vi "11_jednoduchy_trigger.vi"() -> ()   [LabVIEW 2019]
panel:
  in  "Reset Trigger":bool
  out "Hold Trigger":bool
  out "Once Trigger":bool
  out "Waveform Chart":T1(graph)
  in  "stop":bool
  in  "Aktualni hodnota (V)":dbl
  in  "Trigger hodnota (V)":dbl
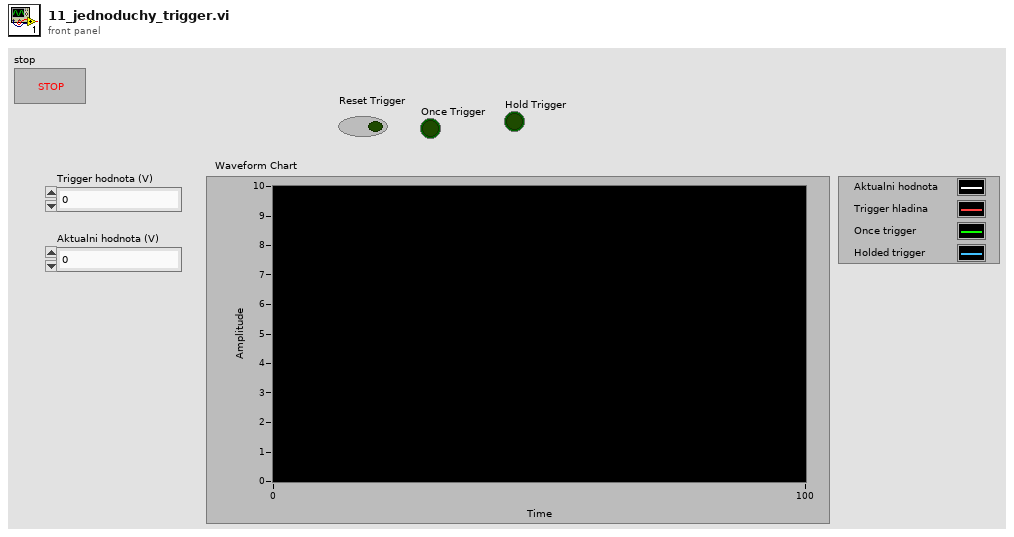
[diagram p1: front panel]
types:
  T1 = cluster{"Aktualni hodnota (V)":dbl, "Trigger hodnota (V)":dbl, i16, i16}
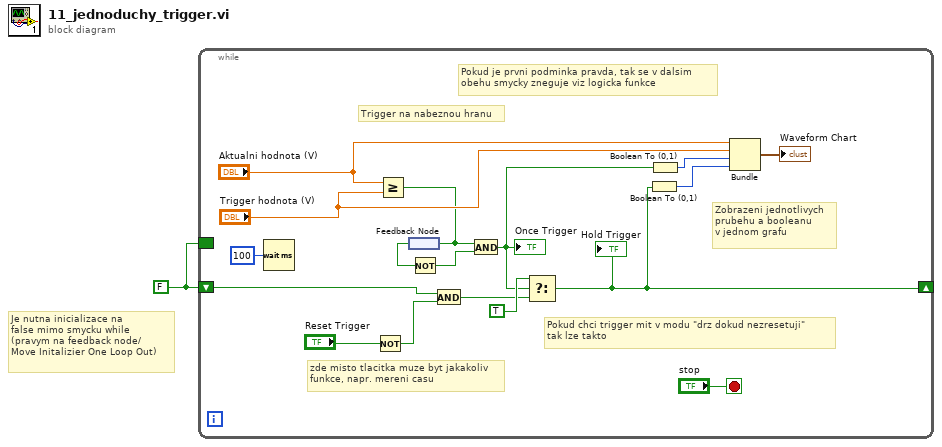
[diagram p0: block diagram]
diagram:
  w1 = FALSE
  # "Je nutna inicializace na\nfalse mimo smycku while\n(pravym na feedback node/\nMove Initalizier One Loop Out)"
  n1 = while {
    shift-right: [w6] -> _
    shift-left: w1 -> [w8]
    border: w1 -> [_]
    stop <- "stop" stop-if-true
    # "zde misto tlacitka muze byt jakakoliv\nfunkce, napr. mereni casu"
    # "Zobrazeni jednotlivych\nprubehu a booleanu\nv jednom grafu"
    # "Pokud chci trigger mit v modu \"drz dokud nezresetuji\"\ntak lze takto"
    # "Pokud je prvni podminka pravda, tak se v dalsim\nobehu smycky zneguje viz logicka funkce"
    # "Trigger na nabeznou hranu"
    n2 = Wait (ms)(milliseconds to wait=u32 100) -> ()  [unwired: 1 out]
    n3 = Not(x="Reset Trigger") -> (.not. x?=w2:bool)
    n4 = Greater Or Equal?(x="Aktualni hodnota (V)", y="Trigger hodnota (V)") -> (x >= y?=w11:bool)
    n5 = feedback-in #1(w11) -> ()
    n6 = feedback #1() -> (w13:bool)
    n7 = Not(x=w13) -> (.not. x?=w12:bool)
    n8 = And(x=w8, y=w2) -> (x .and. y?=w7:bool)
    n9 = And(x=w11, y=w12) -> (x .and. y?=w3:bool)
    "Once Trigger" <- w3
    n10 = Select(t=TRUE, s=w3, f=w7) -> (s? t:f=w6:bool)
    "Hold Trigger" <- w6
    n11 = Boolean To (0,1)(Boolean=w6) -> (0, 1=w4:i16)
    n12 = Boolean To (0,1)(Boolean=w3) -> (0, 1=w5:i16)
    n13 = Bundle("Aktualni hodnota (V)"="Aktualni hodnota (V)", "Trigger hodnota (V)"="Trigger hodnota (V)", w5, w4) -> (→"Waveform Chart":T1)  [unwired: 1 in]
  }
